vi "Change Setpoint.vi"(8 "error in":errorcluster, 10 "Setpoint":dbl format="%#_13g", 11 "Meerstetter TEC in":refnum<class "Meerstetter TEC.lvclass">) -> (0 "error out":errorcluster, 3 "Meerstetter TEC out":refnum<class "Meerstetter TEC.lvclass">)   [LabVIEW 2014, in "Meerstetter Lib.lvlib" / "Meerstetter TEC.lvclass"]
uses:
  Meerstetter TEC.lvclass
  Meerstetter TEC.lvclass/Meerstetter TEC.ctl
  Configurable Device/Configurable Device.lvclass/Configurable Device.ctl
  Configurable Device/Read Log Session.vi
  Configurable Device/Read ID.vi
  Accessors/Write Setpoint.vi
  <userlib>/_Session Fwk/Session - Root.lvclass
  reusable/Session APIs/Session Log/System Log.lvclass
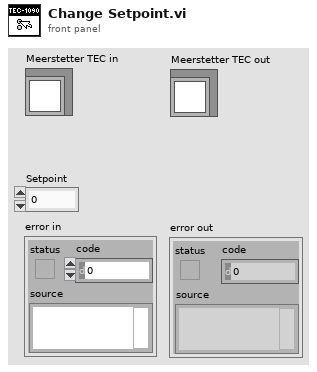
[diagram p1: front panel]
types:
  T1 = typedef "Ctl Method.ctl" = enum16{"Temperature", "Power"}
  T2 = typedef "Session - Root.lvclass/Session Handle.ctl" = refnum<data-value>
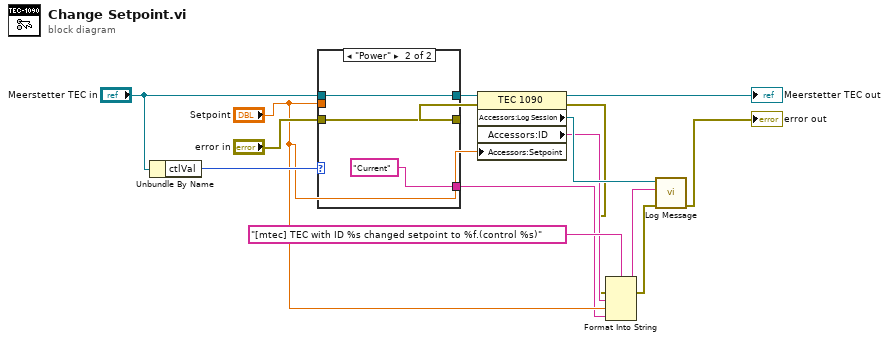
[diagram p0: block diagram]
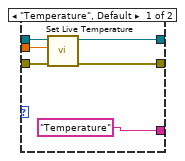
[diagram p2: hidden frame]
diagram:
  n1 = Unbundle By Name("Meerstetter TEC in") -> ("ctlVal"=w15:T1)
  n2 = case shown="\"Power\"" w15 {
    tunnel: "Meerstetter TEC in" -> [w21 w24]
    tunnel: "Setpoint" -> [w19 _]
    tunnel: [w20 w24] -> w12
    tunnel: "error in" -> [w18 w23]
    tunnel: [w17 w23] -> w11
    tunnel: ["Temperature" "Current"] -> w1
    frame "Temperature", Default {
      n3 = call "Set Live Temperature.vi"("error in"=w18, "T"=w19, "TEC 1090 in"=w21) -> ("error out"=w17:errorcluster, "TEC 1090 out"=w20:refnum<class "Meerstetter TEC.lvclass">)  [unwired: 7 in]
    }
    frame "Power" {
    }
  }
  n4 = property class="TEC 1090"(reference=w12, error in=w11, "Accessors:Setpoint"="Setpoint") -> (reference out=→"Meerstetter TEC out":refnum<class "Meerstetter TEC.lvclass">, error out=w5:errorcluster, "Accessors:Log Session"=w9:T2, "Accessors:ID"=w6:string)
  n5 = Format Into String(format string="[mtec] TEC with ID %s changed setpoint to %f.(control %s)", error in=w5, w6, "Setpoint", w1) -> (resulting string=w3:string, error out=w4:errorcluster)  [unwired: 1 in]
  n6 = call "Log Message.vi"("error in"=w4, "MSG In"=w3, "session in"=w9) -> ("error out"=→"error out":errorcluster)  [unwired: 7 in, 1 out]
